vi "Get Stack Info.vi"(8 "error in (no error)":errorcluster, 11 "TIFF in":refnum<class "TIFF.lvclass">) -> (0 "error out":errorcluster, 3 "TIFF out":refnum<class "TIFF.lvclass">)   [LabVIEW 2018, in "BinaryTIFF.lvlib" / "TIFF.lvclass"]
uses:
  TIFF.lvclass
  TIFF.lvclass/TIFF.ctl
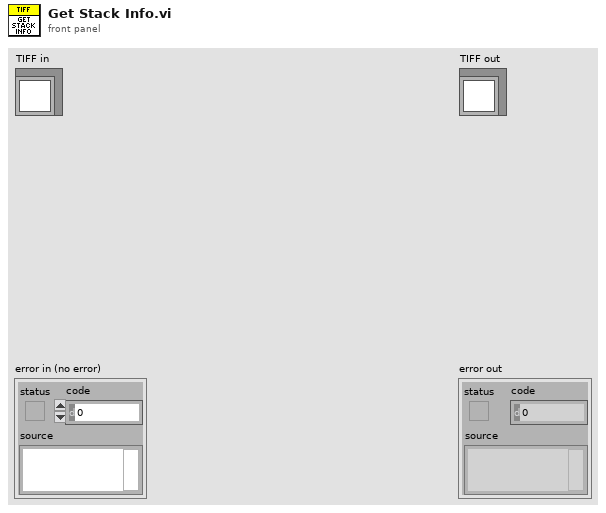
[diagram p1: front panel]
types:
  T1 = cluster{"Offset":u64, "Number of Entries":u64, "IFD Entries":cluster{"Tag":u16, "Data Type":u16, "Number of Elements":u64, "Data":variant}[]}[]
  T2 = cluster{"Offset":u64, "Number of Entries":u64, "IFD Entries":cluster{"Tag":u16, "Data Type":u16, "Number of Elements":u64, "Data":variant}[]}
  T3 = cluster{"Tag":u16, "Data Type":u16, "Number of Elements":u64, "Data":variant}[]
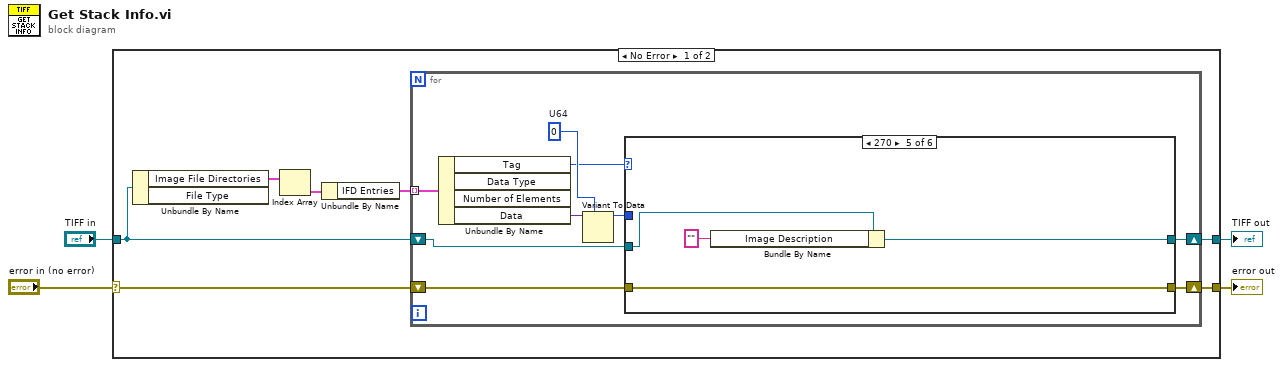
[diagram p0: block diagram]
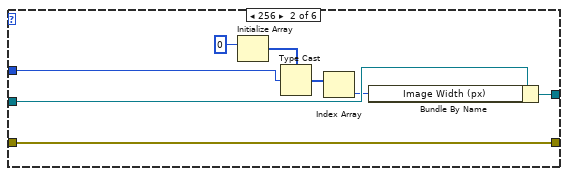
[diagram p3: hidden frame]
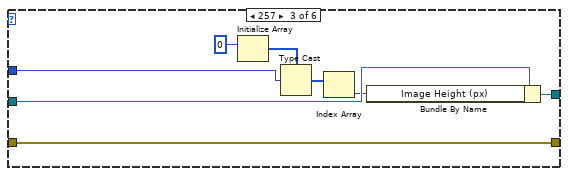
[diagram p4: hidden frame]
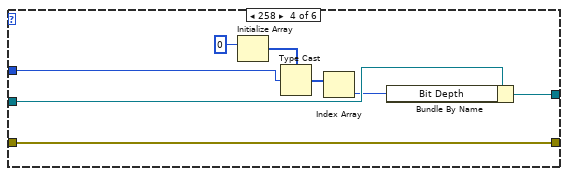
[diagram p5: hidden frame]
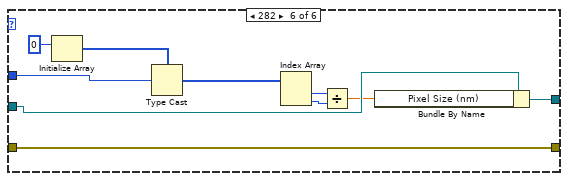
[diagram p6: hidden frame]
diagram:
  n1 = case shown="No Error" "error in (no error)" {
    selector: "error in (no error)" -> [w6 w62]
    tunnel: [w5 w62] -> w3
    tunnel: [w7 w61] -> w1
    tunnel: "TIFF in" -> [w8 w61]
    frame No Error {
      n2 = Unbundle By Name(w8) -> ("Image File Directories"=w11:T1)  [unwired: 1 out]
      n3 = Index Array(array=w11) -> (element=w10:T2)  [unwired: 1 in]
      n4 = Unbundle By Name(w10) -> ("IFD Entries"=w9:T3)
      n5 = for {
        tunnel: w9 -> [w20] mode=indexing
        shift-right: [w18] -> w7
        shift-left: w8 -> [w19]
        shift-right: [w16] -> w5
        shift-left: w6 -> [w17]
        w14 = u64 0  # U64
        n6 = Unbundle By Name(w20) -> ("Tag"=w12:u16, "Data"=w15:variant)  [unwired: 2 out]
        n7 = Variant To Data(type=w14, Variant=w15) -> (data=w13:u64)  [unwired: 1 in, 1 out]
        n8 = case shown="270" w12 {
          tunnel: w19 -> [w22 w30 w38 w46 w50 w59]
          tunnel: [w22 w29 w37 w45 w49 w58] -> w18
          tunnel: w13 -> [_ w24 w32 w42 _ w60]
          tunnel: w17 -> [w21 w28 w36 w44 w48 w51]
          tunnel: [w21 w28 w36 w44 w48 w51] -> w16
          frame 0, Default {
          }
          frame 256 {
            n9 = Initialize Array(u32 0) -> (w26:u32[])  [unwired: 1 in]
            n10 = Type Cast(type=w26, x=w24) -> (*(type *) &x=w25:u32[])
            n11 = Index Array(array=w25) -> (element=w23:u32)  [unwired: 1 in]
            n12 = Bundle By Name(cluster=w30, "Image Width (px)"=w23) -> (w29:refnum<class "TIFF.lvclass">)
          }
          frame 257 {
            n13 = Initialize Array(u32 0) -> (w34:u32[])  [unwired: 1 in]
            n14 = Type Cast(type=w34, x=w32) -> (*(type *) &x=w33:u32[])
            n15 = Index Array(array=w33) -> (element=w31:u32)  [unwired: 1 in]
            n16 = Bundle By Name(cluster=w38, "Image Height (px)"=w31) -> (w37:refnum<class "TIFF.lvclass">)
          }
          frame 258 {
            n17 = Initialize Array(u16 0) -> (w41:u16[])  [unwired: 1 in]
            n18 = Type Cast(type=w41, x=w42) -> (*(type *) &x=w43:u16[])
            n19 = Index Array(array=w43) -> (element=w39:u16)  [unwired: 1 in]
            n20 = Bundle By Name(cluster=w46, "Bit Depth"=w39) -> (w45:refnum<class "TIFF.lvclass">)
          }
          frame 270 {
            n21 = Bundle By Name(cluster=w50, "Image Description"="" ("Stack Info.Image Description")) -> (w49:refnum<class "TIFF.lvclass">)
          }
          frame 282 {
            n22 = Initialize Array(u32 0) -> (w56:u32[])  [unwired: 1 in]
            n23 = Type Cast(type=w56, x=w60) -> (*(type *) &x=w55:u32[])
            n24 = Index Array(array=w55) -> (element #1=w54:u32, element #2=w53:u32)  [unwired: 2 in]
            n25 = Divide(x=w54, y=w53) -> (x/y=w52:dbl)
            n26 = Bundle By Name(cluster=w59, "Pixel Size (nm)"=w52) -> (w58:refnum<class "TIFF.lvclass">)
          }
        }
      }
    }
    frame Error {
    }
  }
  "error out" <- w3
  "TIFF out" <- w1
